vi "2D w X&Y Macro.vi"(0 "2D wave":string, 1 "minimum":dbl, 2 "maximum":dbl, 5 "X wave":string, 7 "Y wave":string, 9 "X,Y,Z Labels":string[](array[string])=["current (nA)", "field (oe)", "dV/dI (Ohm)"], 11 "error in (no error)":errorcluster, 12 "Kill X&Y waves? [T]":bool=TRUE) -> (4 "result string":string, 15 "error out":errorcluster)   [LabVIEW 2019, in "ITX Commands.lvclass"]
uses:
  ITX Commands.lvclass
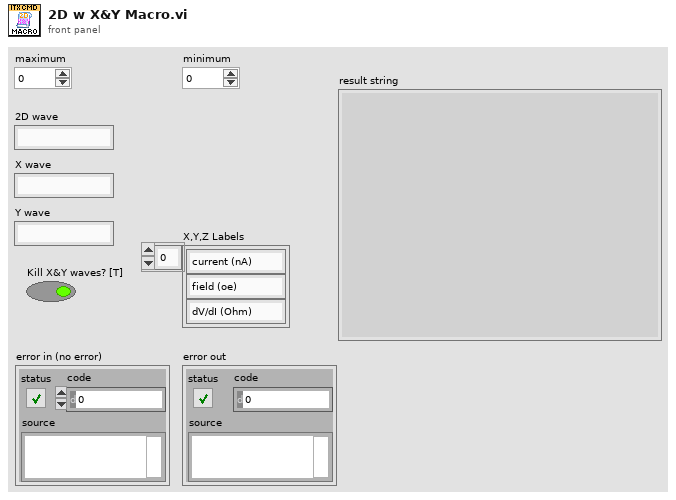
[diagram p1: front panel]
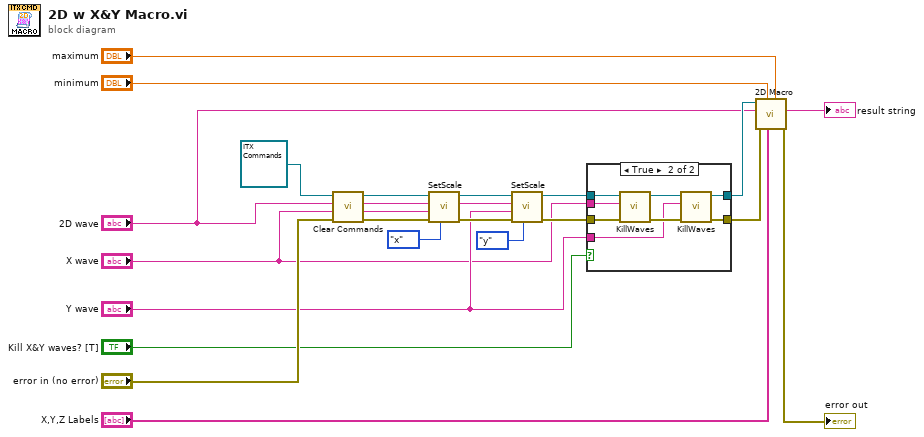
[diagram p0: block diagram]
diagram:
  n1 = call "Clear Commands.vi"("error in (no error)"="error in (no error)", "ITX Commands in"=refnum<class "ITX Commands.lvclass"> refnum) -> ("error out"=w10:errorcluster, "ITX Commands out"=w13:refnum<class "ITX Commands.lvclass">)  [unwired: 8 in]
  n2 = call "SetScale.vi"("Axis"=enum16{"x", "y", "z"}."x", "error in (no error)"=w10, "wavename (Axis)"="X wave", "wavename (Image)"="2D wave", "ITX Commands in"=w13) -> ("error out"=w15:errorcluster, "ITX Commands out"=w14:refnum<class "ITX Commands.lvclass">)  [unwired: 5 in]
  n3 = call "SetScale.vi"("Axis"=enum16{"x", "y", "z"}."y", "error in (no error)"=w15, "wavename (Axis)"="Y wave", "wavename (Image)"="2D wave", "ITX Commands in"=w14) -> ("error out"=w6:errorcluster, "ITX Commands out"=w12:refnum<class "ITX Commands.lvclass">)  [unwired: 5 in]
  n4 = case shown="True" "Kill X&Y waves? [T]" {
    tunnel: w12 -> [w23 w31]
    tunnel: [w23 w28] -> w9
    tunnel: [w22 w27] -> w8
    tunnel: "X wave" -> [_ w26]
    tunnel: w6 -> [w22 w25]
    tunnel: "Y wave" -> [_ w24]
    frame False {
    }
    frame True {
      n5 = call "KillWaves.vi"("error in (no error)"=w25, "wavename"=w26, "ITX Commands in"=w31) -> ("error out"=w29:errorcluster, "ITX Commands out"=w30:refnum<class "ITX Commands.lvclass">)  [unwired: 7 in]
      n6 = call "KillWaves.vi"("error in (no error)"=w29, "wavename"=w24, "ITX Commands in"=w30) -> ("error out"=w27:errorcluster, "ITX Commands out"=w28:refnum<class "ITX Commands.lvclass">)  [unwired: 7 in]
    }
  }
  n7 = call "2D Macro.vi"("maximum"="maximum", "X,Y,Z Labels"="X,Y,Z Labels", "minimum"="minimum", "error in (no error)"=w8, "2D wavename"="2D wave", "ITX Commands in"=w9) -> ("error out"=→"error out":errorcluster, "Commands"=→"result string":string)  [unwired: 3 in, 1 out]
